vi "writeSaveImagesXML.vi"(8 "error in (no error)":errorcluster, 10 "NativeXML in":refnum<class "NativeXML.lvclass">, 11 "PixelflySettings in":refnum<class "PixelflySettings.lvclass">) -> (0 "error out":errorcluster, 2 "NativeXML out":refnum<class "NativeXML.lvclass">, 3 "PixelflySettings out":refnum<class "PixelflySettings.lvclass">)   [LabVIEW 2011, in "Tools.lvlib" / "Settings.lvlib" / "PixelflySettings.lvclass"]
uses:
  PixelflySettings.lvclass
  NativeXML/NativeXML.lvclass
  CamaraSettings.lvclass
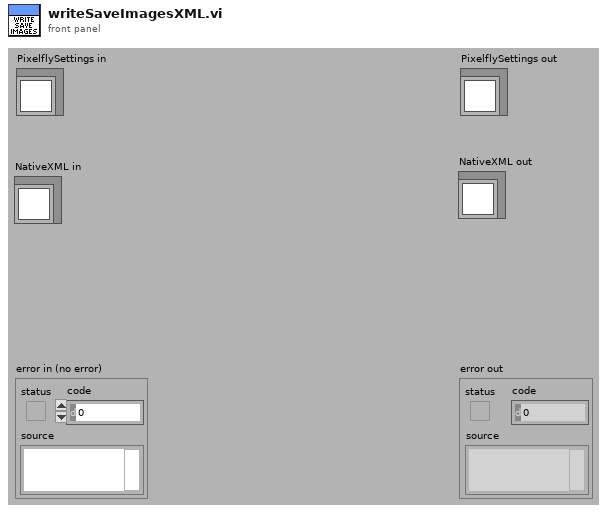
[diagram p1: front panel]
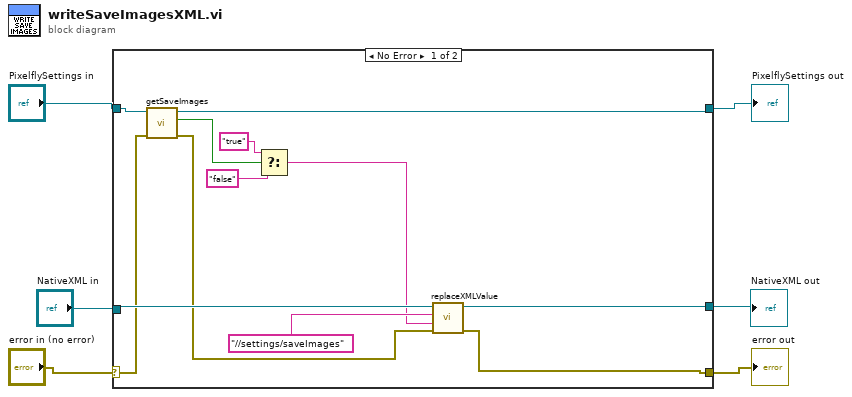
[diagram p0: block diagram]
diagram:
  n1 = case shown="No Error" "error in (no error)" {
    selector: "error in (no error)" -> [w13 w21]
    tunnel: [w15 w21] -> w4
    tunnel: [w7 w20] -> w5
    tunnel: "PixelflySettings in" -> [w14 w20]
    tunnel: "NativeXML in" -> [w18 w19]
    tunnel: [w17 w19] -> w3
    frame No Error {
      n2 = call "getSaveImages.vi"("error in (no error)"=w13, "CamaraSettings in"=w14) -> ("error out"=w12:errorcluster, "saveImages"=w11:bool, "CamaraSettings out"=w7:refnum<class "PixelflySettings.lvclass">)  [unwired: 7 in]
      n3 = Select(t="true", s=w11, f="false") -> (s? t:f=w10:string)
      n4 = call "replaceXMLValue.vi"("error in (no error)"=w12, "value"=w10, "replace in"="//settings/saveImages", "NativeXML in"=w18) -> ("error out"=w15:errorcluster, "NativeXML out"=w17:refnum<class "NativeXML.lvclass">)  [unwired: 6 in]
    }
    frame Error {
    }
  }
  "error out" <- w4
  "PixelflySettings out" <- w5
  "NativeXML out" <- w3
